vi "Pswd creator.vi"() -> ()   [LabVIEW 2012]
uses:
  SubVIs/typedef/User Accounts.ctl
  SubVIs/typedef/User_Data_Cluster.ctl
panel:
  out "Array":T1[](array[typedef])
  out "UD array":string[](array[string])
  out "User-data cluster":T1
  in  "?":T3={"Usuario"="None", "Password"="1234aAaA!", "Account type"=enum."None"}
  in  "?":bool
  in  "file name":string
  out "CypheredText":string
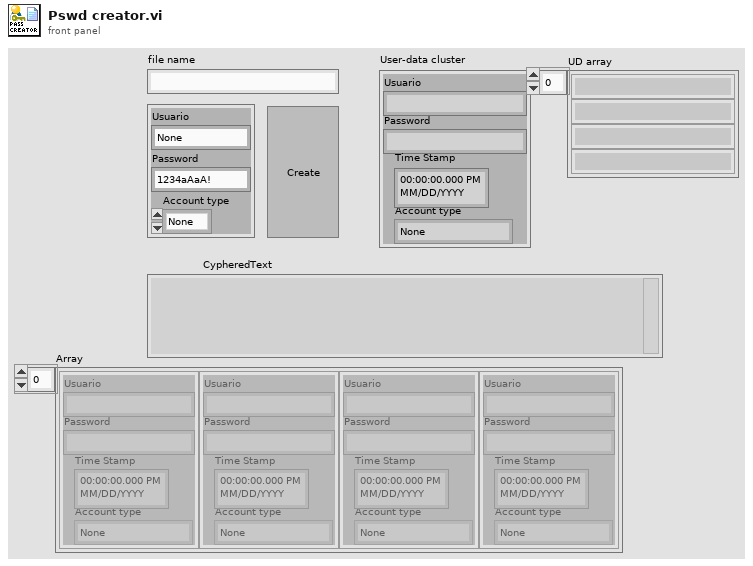
[diagram p1: front panel]
types:
  T1 = typedef "User_Data_Cluster.ctl" = cluster{"Usuario":string, "Password":string, "Account type":T2, "Time Stamp":timestamp}
  T2 = typedef "User Accounts.ctl" = enum16{"None", "User", "Admin"}
  T3 = cluster{"Usuario":string, "Password":string, "Account type":T2}
  T4 = enum16{"open", "replace", "create", "open or create", "replace or create", "replace or create with confirmation"}
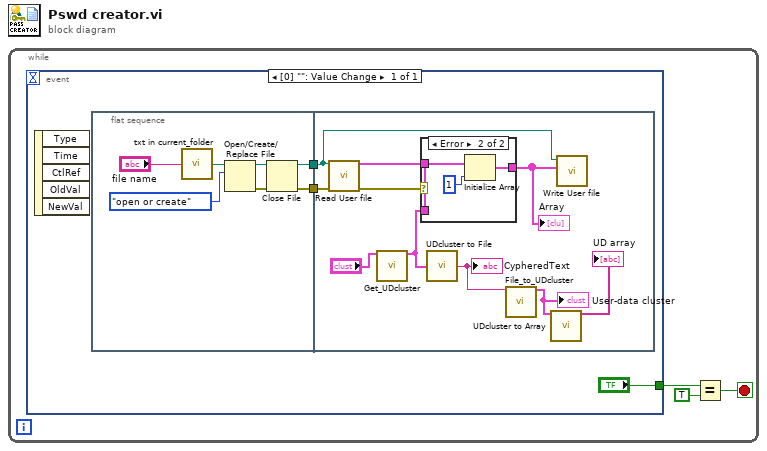
[diagram p0: block diagram]
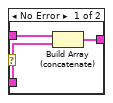
[diagram p2: hidden frame]
diagram:
  n1 = while {
    stop <- w3 stop-if-true
    n2 = event shown="[0] \"\": Value Change" {
      selector: _ -> [_]
      dyn-events: _ -> [_]
      timeout: _ -> [_]
      tunnel: ["?"] -> w1
      event Value Change {
        n3 = event-data() -> ()  [unwired: 1 in, 5 out]
        n4 = flat-sequence {
          tunnel: [w8] -> w5
          tunnel: [w7] -> w4
          tunnel: w5 -> [w22]
          tunnel: w4 -> [w21]
          frame #0 {
            n5 = call "txt in current_folder.vi"("file name"="file name") -> ("Path"=w9:path)  [unwired: 14 in]
            n6 = Open/Create/Replace File(file path (use dialog)=w9, operation (0:open)=T4."open or create") -> (refnum out=w12:refnum<file>, error out=w10:errorcluster)  [unwired: 4 in, 1 out]
            n7 = Close File(refnum=w12, error in=w10) -> (path=w8:path, error out=w7:errorcluster)
          }
          frame #1 {
            n8 = call "Read User file.vi"("file path (use dialog)"=w22, "error in"=w21) -> ("Array"=w23:T1[], "error out"=w20:errorcluster)  [unwired: 12 in]
            n9 = call "Get_UDcluster.vi"("Cluster"="?") -> ("User-data cluster out"=w19:T1)  [unwired: 13 in, 1 out]
            n10 = case shown="Error" w20 {
              tunnel: w23 -> [w26 _]
              tunnel: [w25 w27] -> w14
              tunnel: w19 -> [w24 w28]
              frame No Error {
                n11 = Build Array (concatenate)(w26, w24) -> (w25:T1[])
              }
              frame Error {
                n12 = Initialize Array(w28, 1 ("dimension size")) -> (w27:T1[])
              }
            }
            "Array" <- w14
            n13 = call "UDcluster to File.vi"("User-data cluster"=w19) -> ("CypheredText"=w17:string)
            "CypheredText" <- w17
            n14 = call "File_to_UDcluster.vi"("Cyphered text"=w17) -> ("User-data cluster"=w16:T1)  [unwired: 13 in, 1 out]
            "User-data cluster" <- w16
            n15 = call "UDcluster to Array.vi"("User-data cluster"=w16) -> ("UD array"=→"UD array":string[])  [unwired: 13 in, 1 out]
            n16 = call "Write User file.vi"("Array"=w14, "file path (use dialog)"=w22) -> ()  [unwired: 8 in, 2 out]
          }
        }
      }
    }
    n17 = Equal?(x=w1, y=TRUE) -> (x = y?=w3:bool)
  }
